vi "Adapt Waveform.vi"(8 "Error":errorcluster, 9 "Waveform":T1, 11 "WavBuf":refnum<class "WavBuf.lvclass">) -> (0 "Error Out":errorcluster, 1 "Waveform Out":T1, 3 "WavBuf Out":refnum<class "WavBuf.lvclass">, 5 "Left over Count":i32)   [LabVIEW 2024, in "WavBuf.lvclass"]
uses:
  WavBuf.lvclass
  Universal Controls/Waveform_Data.ctl
  WavBuf.lvclass/WavBuf.ctl
  Support/Measure_Decimate Dbl Array.vi
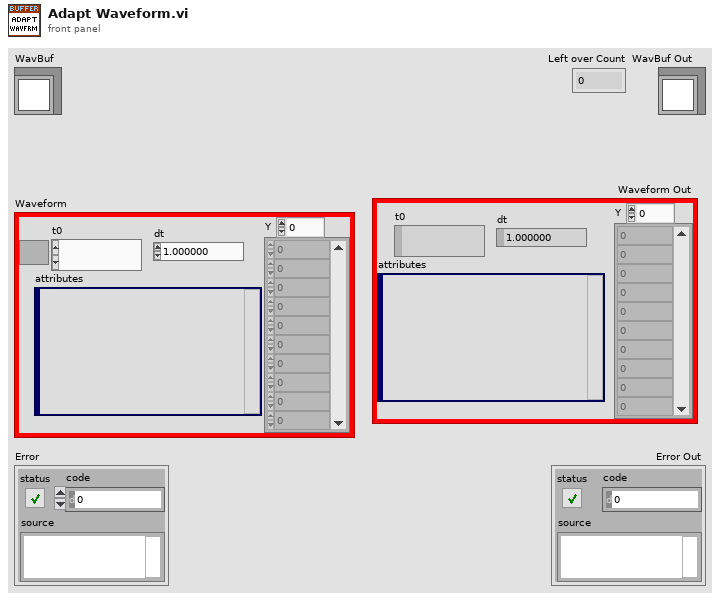
[diagram p1: front panel]
types:
  T1 = typedef "Waveform_Data.ctl" = waveform(dbl)
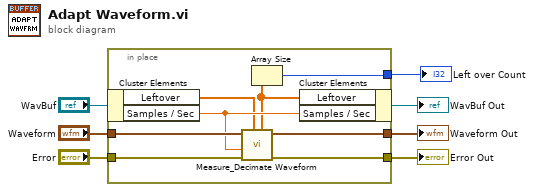
[diagram p0: block diagram]
diagram:
  n1 = in-place {
    in-place-border: [w8] -> w7
    in-place-border: [w11] -> w6
    in-place-border: "Waveform" -> [w15]
    in-place-border: "Error" -> [w12]
    in-place-border: [w9] -> w1
    n2 = in-place-cluster #1("WavBuf") -> ("Leftover"=w13:dbl[], "Samples / Sec"=w14:dbl)
    n3 = call "Measure_Decimate Waveform.vi"("Leftover last"=w13, "Error"=w12, "Target Sample Rate"=w14, "Waveform To Decimate"=w15) -> ("Error Out"=w11:errorcluster, "Waveform Out"=w8:T1, "Leftover Out"=w10:dbl[])  [unwired: 5 in]
    n4 = Array Size(array=w10) -> (size(s)=w9:i32)
    n5 = in-place-cluster #1("Leftover"=w10, "Samples / Sec"=w14) -> (→"WavBuf Out":refnum<class "WavBuf.lvclass">)
  }
  "Waveform Out" <- w7
  "Error Out" <- w6
  "Left over Count" <- w1
